vi "handle_connection.vi"(6 "hangup?":refnum<notifier>, 8 "error in (no error)":errorcluster, 10 "WebSocket Connection":refnum<class "WebSocket Connection.lvclass">, 11 "WebSocket Echo Server in":refnum<class "WebSocket Echo Server.lvclass">) -> (0 "error out":errorcluster)   [LabVIEW 2019, in "WebSocket Echo Server.lvlib" / "WebSocket Echo Server.lvclass"]
uses:
  WebSocket Echo Server.lvclass
  WebSocket Server Toolkit/types/status_code.ctl
  WebSocket Server Toolkit/classes/WebSocket Connection/WebSocket Connection.lvclass
  WebSocket Server Toolkit/WebSocket Server Toolkit.lvlib
panel:
  # "Handle messsages from the receive queue.\nSend messages on the send queue.\nReturn from the VI to hang-up the connection."
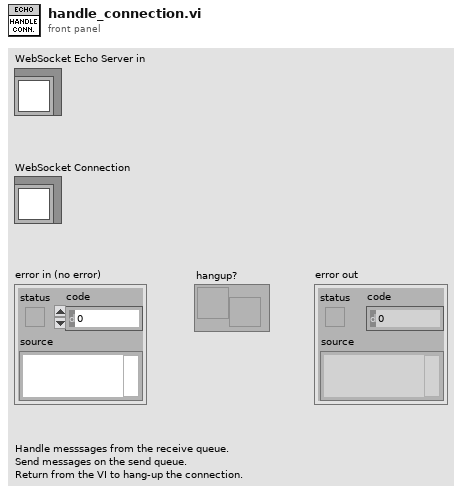
[diagram p1: front panel]
types:
  T1 = typedef "WebSocket Server Toolkit.lvlib/status_code.ctl" = u16
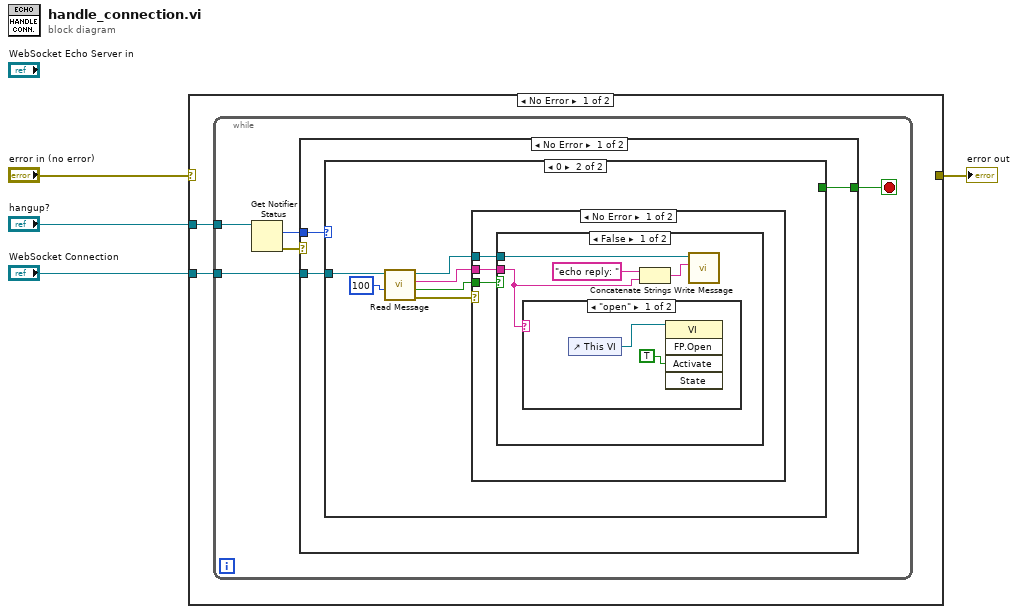
[diagram p0: block diagram]
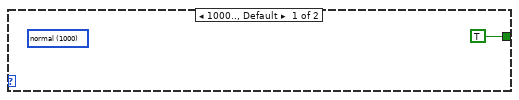
[diagram p2: hidden frame]
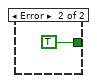
[diagram p6: hidden frame]
diagram:
  n1 = case shown="No Error" "error in (no error)" {
    selector: "error in (no error)" -> [_ w32]
    tunnel: [_ w32] -> w3
    tunnel: "hangup?" -> [w6 _]
    tunnel: "WebSocket Connection" -> [w5 _]
    frame No Error {
      n2 = while {
        tunnel: w6 -> [w11]
        tunnel: w5 -> [w7]
        stop <- w8 stop-if-true
        n3 = Get Notifier Status(notifier=w11) -> (current notification=w9:T1, error out=w10:errorcluster)  [unwired: 1 in, 3 out]
        n4 = case shown="No Error" w10 {
          tunnel: w9 -> [w14 _]
          tunnel: [w13 TRUE] -> w8
          tunnel: w7 -> [w12 _]
          frame No Error {
            n5 = case shown="0" w14 {
              tunnel: [TRUE _] -> w13
              tunnel: w12 -> [_ w21]
              frame 1000.., Default {
                (unwired) T1 1000 items=["ignore"=0, "normal"=1000, "going away"=1001, "protocol error"=1002, "invalid data"=1003] ("latest notification")
              }
              frame 0 {
                n6 = call "Read Message.vi"("timeout in ms (-1)"=100, "WebSocket Connection in"=w21) -> ("error out"=w17:errorcluster, "timed out?"=w16:bool, "message"=w18:string, "WebSocket Connection out"=w19:refnum<class "WebSocket Connection.lvclass">)  [unwired: 5 in, 1 out]
                n7 = case shown="No Error" w17 {
                  tunnel: w16 -> [w24 _]
                  tunnel: w19 -> [w23 _]
                  tunnel: w18 -> [w22 _]
                  frame No Error {
                    n8 = case shown="False" w24 {
                      tunnel: w23 -> [w26 _]
                      tunnel: w22 -> [w25 _]
                      frame False {
                        n9 = case shown="\"open\"" w25 {
                          frame "open" {
                            n10 = control-ref of="This VI"() -> (w30:refnum<vi>)
                            n11 = invoke class="VI" method="FP.Open"(reference=w30, "Activate"=TRUE ("Activate?")) -> ()  [unwired: 3 in, 5 out]
                          }
                          frame Default {
                          }
                        }
                        n12 = Concatenate Strings("echo reply: " ("string"), w25) -> (w27:string)
                        n13 = call "Write Message.vi"("message"=w27, "WebSocket Connection in"=w26) -> ()  [unwired: 8 in, 2 out]
                      }
                      frame True {
                      }
                    }
                  }
                  frame Error {
                  }
                }
              }
            }
          }
          frame Error {
          }
        }
      }
    }
    frame Error {
    }
  }
  "error out" <- w3
